vi "02Manejo_panel 307.vi"(0 "Config Equipos":T2(array[cluster]) {"Ref PD" max=10000 step=1; "Med Princ" items=["1", "2", "3", "4", "5", "6", "7", "8", "9", "10", "11", "12", "13", "14", "15", "16", "17", "18", "19", "20", "21", "22", "23", "24", "25", "26", "27", "28", "29", "30", "31", "32"]}, 1 "Med nº":u8, 2 "Mediciones":T1, 3 "Nº equipo":i32, 4 "Paneles in":T4(array[cluster]) {"Nº" min=1.0 max=60.0 step=1.0 format="%#2.1f"; "Ultima recepción" format="%<%d/%m - %X>T"; "Med\nPpal" format="%_4g"}) -> (5 "Paneles out":T3(array[cluster]) {"Numeric" min=1.0 max=60.0 step=1.0 format="%#2.1f"; "Ultima recepción" format="%<%d/%m - %X>T"; "Med\nPpal" format="%_4g"})   [LabVIEW 2010]
panel:
  in  "Flags recep":bool[](array[boolean])
  out "T. error":timestamp[](array[timestamp])
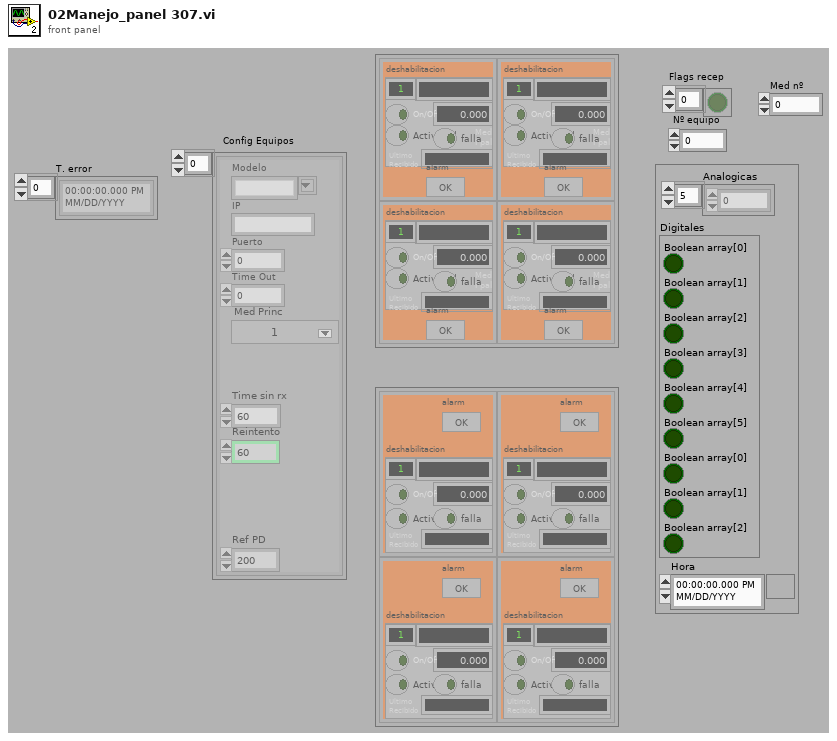
[diagram p1: front panel]
types:
  T1 = cluster{"Analogicas":sgl[], "Digitales":cluster{"Boolean array[0]":bool, "Boolean array[1]":bool, "Boolean array[2]":bool, "Boolean array[3]":bool, "Boolean array[4]":bool, "Boolean array[5]":bool, "Boolean array[0]":bool, "Boolean array[1]":bool, "Boolean array[2]":bool}, "Hora":timestamp}
  T2 = cluster{"Modelo":string, "IP":string, "Puerto":u16, "Time Out":u16, "Med Princ":u16, "Time sin rx":u16, "Reintento":u16, "Ref PD":u16}[]
  T3 = cluster{"Nombre":string, "Med\nPpal":dbl, "On/Off":bool, "Ultima recepción":timestamp, "Numeric":dbl, "deshabilitacion":bool, "Actividad":bool, "falla":bool, "alarm":bool}[][]
  T4 = cluster{"Nombre":string, "Med\nPpal":dbl, "On/Off":bool, "Ultima recepción":timestamp, "Nº":dbl, "deshabilitacion":bool, "Actividad":bool, "falla":bool, "alarm":bool}[][]
  T5 = cluster{"Boolean array[0]":bool, "Boolean array[1]":bool, "Boolean array[2]":bool, "Boolean array[3]":bool, "Boolean array[4]":bool, "Boolean array[5]":bool, "Boolean array[0]":bool, "Boolean array[1]":bool, "Boolean array[2]":bool}
  T6 = cluster{"Modelo":string, "IP":string, "Puerto":u16, "Time Out":u16, "Med Princ":u16, "Time sin rx":u16, "Reintento":u16, "Ref PD":u16}
  T7 = cluster{"Boolean array[0]":bool, "Boolean array[1]":bool, "Boolean array[2]":bool, "Boolean array[2]":bool, "Boolean array[4]":bool, "Boolean array[4]":bool, "Boolean array[4]":bool, "Boolean array[4]":bool, "Boolean array[4]":bool, "Boolean array[4]":bool, "Boolean array[4]":bool}
  T8 = cluster{"Nombre":string, "Med\nPpal":dbl, "On/Off":bool, "Ultima recepción":timestamp, "Nº":dbl, "deshabilitacion":bool, "Actividad":bool, "falla":bool, "alarm":bool}
  T9 = cluster{"Nombre":string, "Numeric":sgl, "On/Off":bool, "Ultima recepción":timestamp, "Nº":dbl, "deshabilitacion":bool, bool, bool, bool}
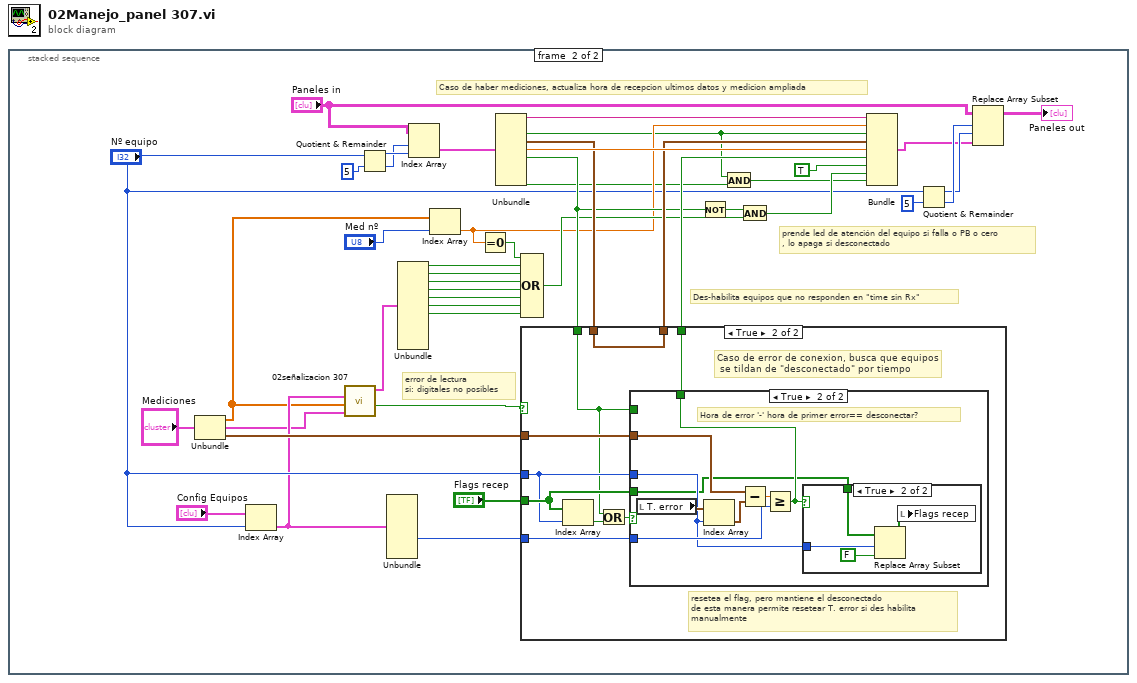
[diagram p0: block diagram]
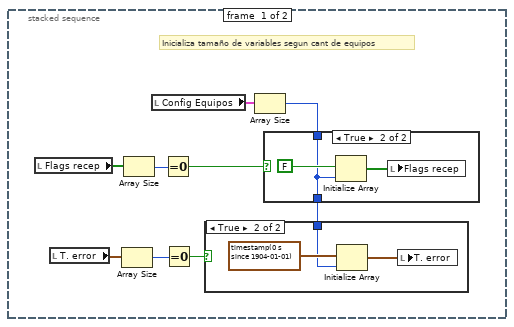
[diagram p2: hidden frame]
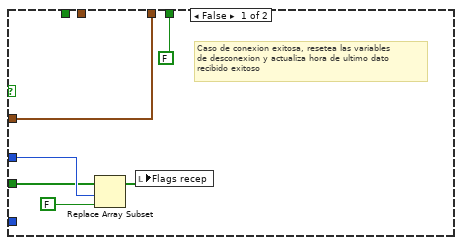
[diagram p5: hidden frame]
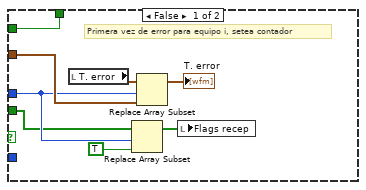
[diagram p6: hidden frame]
diagram:
  n1 = stacked-sequence {
    frame #0 {
      # "Inicializa tamaño de variables segun cant de equipos"
      n2 = local read "Flags recep"() -> (w9:bool[])
      n3 = local read "T. error"() -> (w8:timestamp[])
      n4 = Array Size(array=w8) -> (size(s)=w4:i32)
      n5 = Array Size(array=w9) -> (size(s)=w7:i32)
      n6 = local read "Config Equipos"() -> (w3:T2)
      n7 = Equal To 0?(x=w7) -> (x = 0?=w6:bool)
      n8 = Equal To 0?(x=w4) -> (x = 0?=w5:bool)
      n9 = Array Size(array=w3) -> (size(s)=w2:i32)
      n10 = case shown="True" w6 {
        tunnel: w2 -> [w13 w14]
        tunnel: [w13 w14] -> w1
        frame False {
        }
        frame True {
          n11 = Initialize Array(FALSE, w14) -> (w16:bool[])
          n12 = local write "Flags recep"(w16) -> ()
        }
      }
      n13 = case shown="True" w5 {
        tunnel: w1 -> [_ w10]
        frame False {
        }
        frame True {
          n14 = Initialize Array(timestamp(0 s since 1904-01-01), w10) -> (w12:timestamp[])
          n15 = local write "T. error"(w12) -> ()
        }
      }
    }
    frame #1 {
      # "error de lectura\nsi: digitales no posibles"
      # "prende led de atención del equipo si falla o PB o cero\n, lo apaga si desconectado"
      # "Des-habilita equipos que no responden en \"time sin Rx\""
      # "Caso de haber mediciones, actualiza hora de recepcion ultimos datos y medicion ampliada"
      n16 = Unbundle("Mediciones") -> ("Analogicas"=w27:sgl[], "Digitales"=w26:T5, "Hora"=w52:timestamp)
      n17 = Index Array(array="Config Equipos", index="Nº equipo") -> (element=w28:T6)
      n18 = call "02señalizacion 307.vi"("Digitales"=w26, "Analogicas"=w27, "Config Equipo"=w28) -> ("error lectura"=w25:bool, "Señalizacion"=w24:T7)  [unwired: 1 in, 2 out]
      n19 = Quotient & Remainder(x="Nº equipo", y=5) -> (x-y*floor(x/y)=w37:i32, floor(x/y)=w36:i32)
      n20 = Unbundle(w28) -> ("Time sin rx"=w53:u16)  [unwired: 7 out]
      n21 = Unbundle(w24) -> ("Boolean array[0]"=w23:bool, "Boolean array[1]"=w22:bool, "Boolean array[2]"=w21:bool, "Boolean array[2]"=w20:bool, "Boolean array[4]"=w19:bool, "Boolean array[4]"=w18:bool, "Boolean array[4]"=w17:bool)  [unwired: 4 out]
      n22 = Index Array(array="Paneles in", index (row)=w36, index (col)=w37) -> (element=w35:T8)
      n23 = Index Array(array=w27, index="Med nº") -> (element=w47:sgl)
      n24 = Equal To 0?(x=w47) -> (x = 0?=w46:bool)
      n25 = Unbundle(w35) -> ("Nombre"=w59:string, "On/Off"=w31:bool, "Ultima recepción"=w57:timestamp, "Nº"=w60:dbl, "deshabilitacion"=w51:bool, "alarm"=w30:bool)  [unwired: 3 out]
      n26 = Compound Arithmetic op=OR(w46, w23, w22, w21, w20, w19, w18, w17) -> (w48:bool)
      n27 = case shown="True" w25 {
        tunnel: w52 -> [w66 w74]
        tunnel: [w66 w75] -> w58
        tunnel: w57 -> [_ w75]
        tunnel: w53 -> [_ w73]
        tunnel: "Nº equipo" -> [w63 w71]
        tunnel: "Flags recep" -> [w62 w72]
        tunnel: w51 -> [_ w67]
        tunnel: [FALSE ("new element/subarray") w69] -> w55
        frame False {
          # "Caso de conexion exitosa, resetea las variables\nde desconexion y actualiza hora de ultimo dato\nrecibido exitoso"
          n28 = Replace Array Subset(array=w62, new element=FALSE ("new element/subarray"), index=w63) -> (w65:bool[])
          n29 = local write "Flags recep"(w65) -> ()
        }
        frame True {
          # "resetea el flag, pero mantiene el desconectado\nde esta manera permite resetear T. error si des habilita\nmanualmente"
          # "Caso de error de conexion, busca que equipos\n se tildan de \"desconectado\" por tiempo"
          n30 = Index Array(array=w72, index=w71) -> (element=w68:bool)
          n31 = Or(x=w67, y=w68) -> (x .or. y?=w70:bool)
          n32 = case shown="True" w70 {
            tunnel: w74 -> [w79 w91]
            tunnel: w73 -> [_ w87]
            tunnel: w71 -> [w78 w86]
            tunnel: w72 -> [w77 w84]
            tunnel: w67 -> [w76 _]
            tunnel: [w76 w85] -> w69
            frame False {
              # "Primera vez de error para equipo i, setea contador"
              n33 = local read "T. error"() -> (w83:timestamp[])
              n34 = Replace Array Subset(array=w77, new element=TRUE ("new element/subarray"), index=w78) -> (w81:bool[])
              n35 = Replace Array Subset(array=w83, new element=w79, index=w78) -> (→"T. error":timestamp[])
              n36 = local write "Flags recep"(w81) -> ()
            }
            frame True {
              # "Hora de error '-' hora de primer error== desconectar?"
              n37 = local read "T. error"() -> (w90:timestamp[])
              n38 = Index Array(array=w90, index=w86) -> (element=w89:timestamp)
              n39 = Subtract(x=w91, y=w89) -> (x-y=w88:dbl)
              n40 = Greater Or Equal?(x=w88, y=w87) -> (x >= y?=w85:bool)
              n41 = case shown="True" w85 {
                tunnel: w86 -> [_ w94]
                tunnel: w84 -> [_ w92]
                frame False {
                }
                frame True {
                  n42 = Replace Array Subset(array=w92, new element=FALSE ("new element/subarray"), index=w94) -> (w95:bool[])
                  n43 = local write "Flags recep"(w95) -> ()
                }
              }
            }
          }
        }
      }
      n44 = Not(x=w51) -> (.not. x?=w49:bool)
      n45 = And(x=w31, y=w30) -> (x .and. y?=w32:bool)
      n46 = And(x=w49, y=w48) -> (x .and. y?=w50:bool)
      n47 = Bundle("Nombre"=w59, "Numeric"=w47, "On/Off"=w31, "Ultima recepción"=w58, "Nº"=w60, "deshabilitacion"=w55, TRUE, w50, w32) -> (w39:T9)  [unwired: 1 out]
      n48 = Quotient & Remainder(x="Nº equipo", y=5) -> (x-y*floor(x/y)=w42:i32, floor(x/y)=w43:i32)
      n49 = Replace Array Subset(array="Paneles in", new element=w39, index (row)=w43, index (col)=w42) -> (→"Paneles out":T4)
    }
  }
